vi "Define Domain.vi"(5 "target Domain":refnum<class "NI_Domain.lvclass">, 7 "target PDE":refnum<class "NI_PDE.lvclass">, 8 "error in (no error)":errorcluster, 10 "domain":variant, 11 "PDE in":refnum<class "NI_PDE.lvclass">) -> (0 "error out":errorcluster, 3 "PDE out":refnum<class "NI_PDE.lvclass">)   [LabVIEW 2017, in "NI_PDE.lvlib" / "NI_PDE.lvclass"]
uses:
  <vilib>/gmath/pde.llb/PDEClass/NI_PDE.lvclass
  <vilib>/gmath/pde.llb/DomainClass/NI_Domain.lvclass
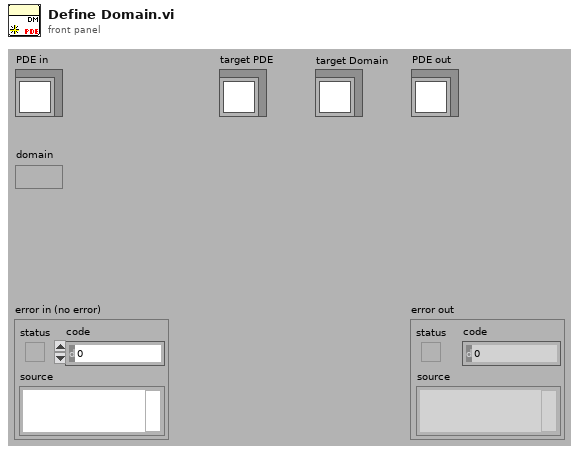
[diagram p1: front panel]
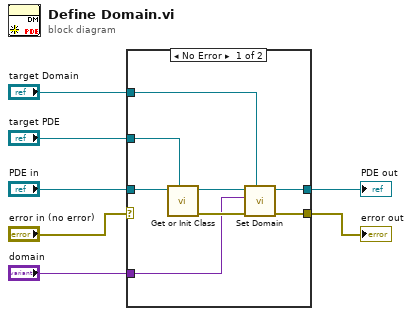
[diagram p0: block diagram]
diagram:
  n1 = case shown="No Error" "error in (no error)" {
    selector: "error in (no error)" -> [_ w17]
    tunnel: "PDE in" -> [w11 w16]
    tunnel: [w13 w16] -> w7
    tunnel: [w12 w17] -> w6
    tunnel: "target Domain" -> [w9 _]
    tunnel: "target PDE" -> [w8 _]
    tunnel: "domain" -> [w10 _]
    frame No Error {
      n2 = call <vilib>:"Get or Init Class.vi"("target PDE"=w8, "PDE in"=w11) -> ("error out"=w14:errorcluster, "PDE out"=w15:refnum<class "NI_PDE.lvclass">)  [unwired: 2 in, 6 out]
      n3 = call <vilib>:"Set Domain.vi"("target Domain"=w9, "error in (no error)"=w14, "domain"=w10, "PDE in"=w15) -> ("error out"=w12:errorcluster, "PDE out"=w13:refnum<class "NI_PDE.lvclass">)  [unwired: 6 out]
    }
    frame Error {
    }
  }
  "PDE out" <- w7
  "error out" <- w6
